vi "_FPGA Load Oscillator.vi"(4 "error in":errorcluster) -> (0 "error out":errorcluster)   [LabVIEW 2012]
uses:
  _RT Global.vi
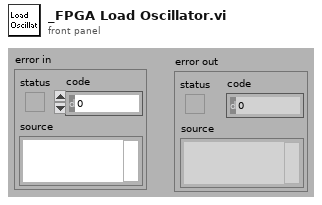
[diagram p1: front panel]
types:
  T1 = typedef "_RT Instrument 2.ctl" = cluster{"Table":T2[], "Instrument":string[]}
  T2 = typedef "_RT Configuration 2.ctl" = cluster{"Name":string, "Ch#":u8, "Min":dbl, "Max":dbl, "Def+":dbl, "Def-":dbl, "Offset":dbl, "Slope":dbl, "Type":u8, "Description":string, "SettleT":dbl}
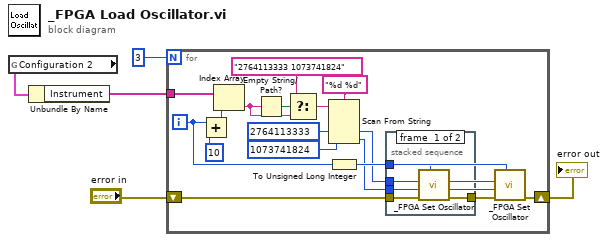
[diagram p0: block diagram]
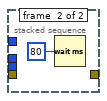
[diagram p2: hidden frame]
diagram:
  n1 = global read "_RT Global.vi" "Configuration 2"() -> (w5:T1)
  n2 = Unbundle By Name(w5) -> ("Instrument"=w2:string[])
  n3 = for {
    N: 3 -> [_]
    tunnel: w2 -> [w22]
    shift-right: [w6] -> w1
    shift-left: "error in" -> [w11]
    i -> [w12]
    n4 = Add(x=w12, y=10) -> (x+y=w20:i32)
    n5 = Index Array(array=w22, index=w20) -> (element=w18:string)
    n6 = Empty String/Path?(string/path=w18) -> (empty?=w19:bool)
    n7 = Select(t="2764113333 1073741824", s=w19, f=w18) -> (s? t:f=w16:string)
    n8 = Scan From String(format string="%d %d", input string=w16, default 1=u32 2764113333 ("default value 1"), default 2=u32 1073741824 ("default value 1")) -> (output 1=w8:u32, output 2=w7:u32)  [unwired: 2 in, 3 out]
    n9 = To Unsigned Long Integer(number=w12) -> (unsigned 32bit integer=w9:u32)
    n10 = stacked-sequence {
      tunnel: w9 -> [w27 _]
      tunnel: w8 -> [w26 _]
      tunnel: w7 -> [w25 _]
      tunnel: w11 -> [w24 _]
      tunnel: [w23 _] -> w10
      frame #0 {
        n11 = call "_FPGA Set Oscillator.vi"("Param 3"=w27, "error in"=w24, "Param 2"=w25, "Param 1"=w26) -> ("error out"=w23:errorcluster)  [unwired: 1 in, 3 out]
      }
      frame #1 {
        n12 = Wait (ms)(milliseconds to wait=u32 80) -> ()  [unwired: 1 out]
      }
    }
    n13 = call "_FPGA Set Oscillator.vi"("Param 3"=w9, "error in"=w10, "Param 2"=w7, "Param 1"=w8) -> ("error out"=w6:errorcluster)  [unwired: 1 in, 3 out]
  }
  "error out" <- w1
